vi "Get Start and Stop Channels.vi"(8 "error in":errorcluster, 11 "terminal":T1 format="%.0x") -> (0 "error out":errorcluster, 1 "stop channel":T1 format="%.0x", 2 "start channel":T1 format="%.0x", 3 "terminal out":T1 format="%.0x", 4 "found?":bool)   [LabVIEW 2020, in "AIM MIL-STD-1553 Scripting.lvlib"]
doc: "Returns the <b>start channel</b> and <b>stop channel</b> for the specified <b>terminal</b>. <b>found?</b> returns False if either of the command channels is missing."
uses:
  AIM MIL-STD-1553 Scripting.lvlib
  <vilib>/NI VeriStand/Custom Device API/Custom Device Item Ref.ctl
  Constants.vi
  <vilib>/NI VeriStand/Custom Device Tools/Custom Device Utility Library/NI VeriStand - Search for Item by Name.vi
  <vilib>/NI VeriStand/Custom Device Tools/Custom Device Utility Library/Custom Device Utility Library.lvlib
  <vilib>/NI VeriStand/Custom Device API/Custom Device API.lvlib
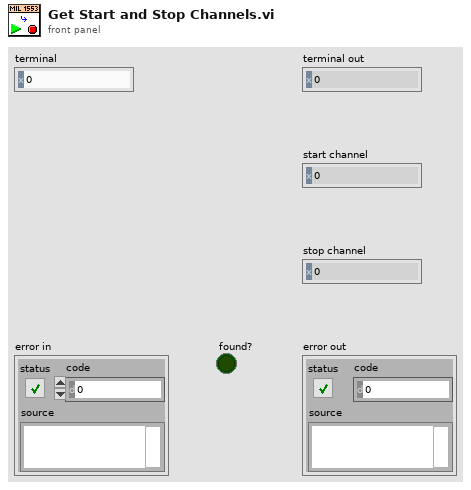
[diagram p1: front panel]
types:
  T1 = typedef "Custom Device API.lvlib/Custom Device Item Ref.ctl" = u64
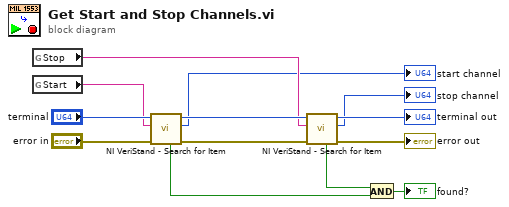
[diagram p0: block diagram]
diagram:
  n1 = global read "Constants.vi" "Stop"() -> (w6:string)
  n2 = global read "Constants.vi" "Start"() -> (w7:string)
  n3 = call-poly <vilib>:"NI VeriStand - Search for Item.vi"("error in"="error in", "Item Name"=w7, "Section Ref in"="terminal") -> ("error out"=w11:errorcluster, "Item Ref"=→"start channel":T1, "Section Ref out"=w12:T1, "Found"=w2:bool)  [unwired: 5 in]
  n4 = call-poly <vilib>:"NI VeriStand - Search for Item.vi"("error in"=w11, "Item Name"=w6, "Section Ref in"=w12) -> ("error out"=→"error out":errorcluster, "Item Ref"=→"stop channel":T1, "Section Ref out"=→"terminal out":T1, "Found"=w3:bool)  [unwired: 5 in]
  n5 = And(x=w3, y=w2) -> (x .and. y?=→"found?":bool)
